vi "Actor Core.vi"(8 "error in":errorcluster, 11 "Server in":refnum<class "Server.lvclass">) -> (0 "error out":errorcluster, 3 "Actor out":refnum<class "Actor.lvclass">)   [LabVIEW 2015, in "Server.lvlib" / "Server.lvclass"]
doc: "(<B>Filename</B>: Actor Framework.lvlib:Actor.lvclass:Actor Core.vi)\n\nReceives messages to the actor, reacts to them, and initiates any error handling that may shut the actor down.\n\nDescendant classes may override this VI to append parallel tasks for the actor to complete while it handles messages. Overrides use the Call Parent Method node."
uses:
  Server.lvclass
  <vilib>/ActorFramework/Actor/Actor.lvclass
  <vilib>/ActorFramework/Stop Msg/Stop Msg.lvclass
  Server Messages/Launch New Chat Window Msg/Launch New Chat Window Msg.lvclass
  Server Messages/Send Global Chat Msg/Send Global Chat Msg.lvclass
panel:
  in  "Send Chat":bool
  in  "Message":string
  in  "Launch Chat Window":bool
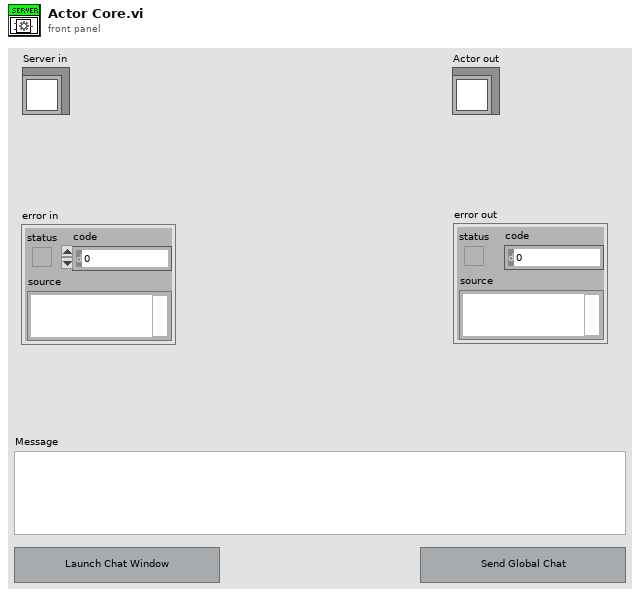
[diagram p1: front panel]
types:
  T1 = enum8{"Enabled", "Disabled", "Disabled and Grayed Out"}
  T2 = enum32{"Invalid", "Standard", "Closed", "Hidden", "Minimized", "Maximized"}
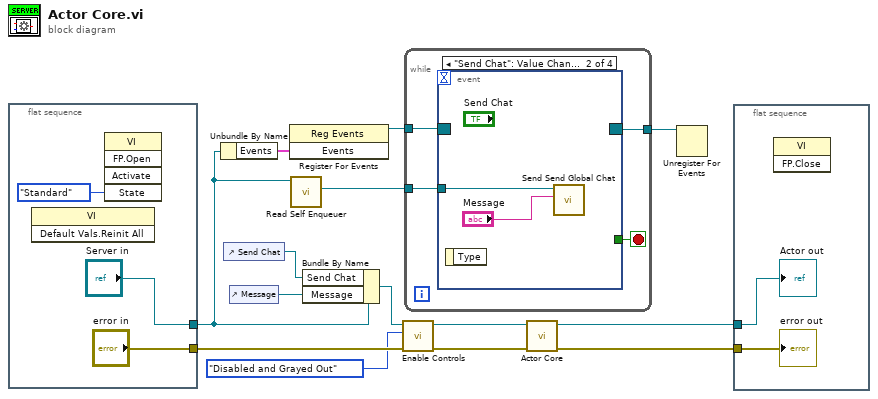
[diagram p0: block diagram]
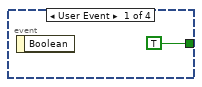
[diagram p2: hidden frame]
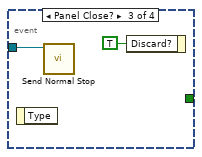
[diagram p3: hidden frame]
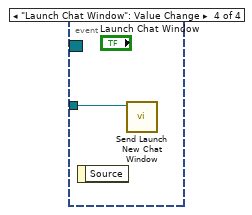
[diagram p4: hidden frame]
diagram:
  n1 = flat-sequence {
    tunnel: ["error in"] -> w12
    tunnel: ["Server in"] -> w7
    frame #0 {
      n2 = invoke class="VI" method="Default Vals.Reinit All"() -> ()  [unwired: 3 in, 3 out]
      n3 = invoke class="VI" method="FP.Open"("State"=T2."Standard") -> ()  [unwired: 4 in, 5 out]
    }
  }
  n4 = Unbundle By Name(w7) -> ("Events"=w11:cluster{"Stop":refnum<user-event>})
  n5 = control-ref of="Send Chat"() -> (w5:refnum<vi>)
  n6 = control-ref of="Message"() -> (w6:refnum<vi>)
  n7 = register-events(w11) -> (reference out=w10:refnum<event-registration>)  [unwired: 2 in, 1 out]
  n8 = call <vilib>:"Read Self Enqueuer.vi"("Actor"=w7) -> ("Self Enqueuer"=w8:refnum<class "Message Enqueuer.lvclass">)  [unwired: 10 in]
  n9 = Bundle By Name(cluster=w7, "Send Chat"=w5, "Message"=w6) -> (w3:refnum<class "Server.lvclass">)
  n10 = call "Enable Controls.vi"("error in (no error)"=w12, "Disabled"=T1."Disabled and Grayed Out", "Server in"=w3) -> ("error out"=w4:errorcluster, "Server out"=w2:refnum<class "Server.lvclass">)  [unwired: 7 in]
  n11 = while {
    tunnel: w10 -> [w21]
    tunnel: [w19] -> w9
    tunnel: w8 -> [w18]
    stop <- w20 stop-if-true
    n12 = event shown="[1] \"Send Chat\": Value Change" {
      selector: w21 -> [_ _ _ _]
      dyn-events: [_ _ _ _] -> w19
      timeout: _ -> [_ _ _ _]
      tunnel: [TRUE _ _ _] -> w20
      tunnel: w18 -> [_ w24 w25 w27]
      event User Event {
        n13 = event-data() -> ()  [unwired: 1 in, 1 out]
      }
      event "Send Chat": Value Change {
        n14 = event-data() -> ()  [unwired: 1 in, 1 out]
        n15 = call "Send Send Global Chat.vi"("Message"="Message", "Message Enqueuer"=w24) -> ()  [unwired: 8 in, 2 out]
      }
      event Panel Close? {
        n16 = event-data() -> ()  [unwired: 1 in, 1 out]
        n17 = call <vilib>:"Send Normal Stop.vi"("Message Enqueuer"=w25) -> ()  [unwired: 10 in, 1 out]
        n18 = event-data("Discard?"=TRUE) -> ()  [unwired: 1 in, 1 out]
      }
      event "Launch Chat Window": Value Change {
        n19 = event-data() -> ()  [unwired: 1 in, 1 out]
        n20 = call "Send Launch New Chat Window.vi"("Message Enqueuer"=w27) -> ()  [unwired: 9 in, 2 out]
      }
    }
  }
  n21 = call-parent "Actor Core.vi"("error in"=w4, "Actor in"=w2) -> ("error out"=w14:errorcluster, "Actor out"=w13:refnum<class "Actor.lvclass">)  [unwired: 8 in]
  n22 = Unregister For Events(event registration refnum=w9) -> ()  [unwired: 1 in, 1 out]
  n23 = flat-sequence {
    tunnel: w14 -> [w29]
    tunnel: w13 -> [w28]
    frame #0 {
      n24 = invoke class="VI" method="FP.Close"() -> ()  [unwired: 3 in, 3 out]
      "error out" <- w29
      "Actor out" <- w28
    }
  }
